vi "DS360 Receive Message.vi"(2 "timeout ms":u32=25000, 3 "address string":string, 4 "byte count":i32, 7 "source":string, 8 "read mode (EOI:0)":i32(ring)=2 items=["terminate read on EOI or byte count", "terminate read on EOI, byte count, or CR", "terminate read on EOI, byte count, or LF"], 9 "error in":T1) -> (0 "address out":string, 1 "read buffer":string, 5 "status":bool[](array[boolean]), 6 "error out":T1)   [LabVIEW 2025, in "MyDS360.lvlib"]
doc: "Sends a string to a message based VXI instrument. In order to communicate with an instrument, you must first open the instrument by running the Open VXI Instrument or running the initialize VI (initialize VIs call the Open VXI Instrument in their block diagram). Use the instrument ID generated by the Open VXI Instrument to address the specific instrument, then set the write mode and enter the string to send. If a write error occurs, error code 1230 is returned. If you fail to open the instrument, error code 1232 is returned."
uses:
  MyDS360.lvlib
panel:
  in  "[empty array]":bool[](array[boolean])
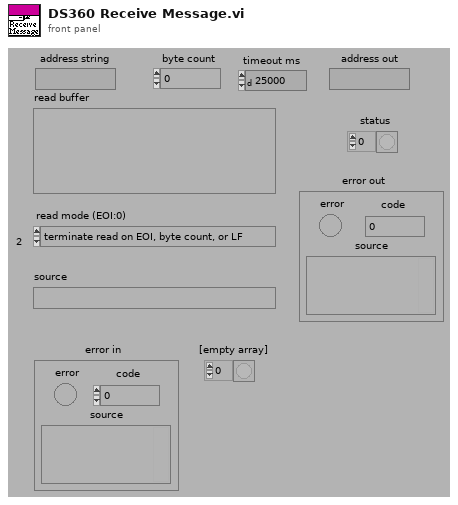
[diagram p1: front panel]
types:
  T1 = cluster{"error":bool, "code":i32, "source":string}
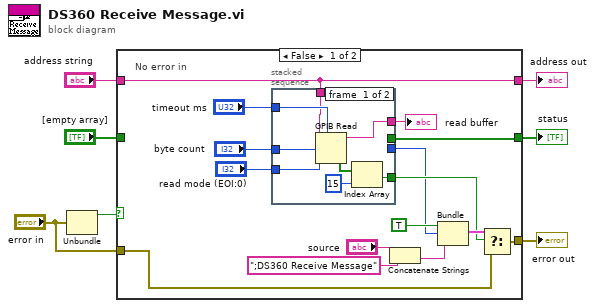
[diagram p0: block diagram]
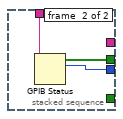
[diagram p2: hidden frame]
diagram:
  n1 = Unbundle("error in") -> ("error"=w5:bool)  [unwired: 2 out]
  n2 = case shown="False" w5 {
    tunnel: "[empty array]" -> [_ w35]
    tunnel: [w18 w35] -> w7
    tunnel: [w21 w36] -> w3
    tunnel: "error in" -> [w13 w36]
    tunnel: "address string" -> [w8 w34]
    tunnel: [w8 w34] -> w1
    frame False {
      # "No error in"
      n3 = stacked-sequence {
        tunnel: [_ w33] -> w18
        tunnel: [w28 _] -> w19
        tunnel: [_ w32] -> w17
        tunnel: "timeout ms" -> [w27 _]
        tunnel: "read mode (EOI:0)" -> [w26 _]
        tunnel: "byte count" -> [w25 _]
        tunnel: [w24 _] -> w9
        tunnel: w8 -> [w23 w31]
        frame #0 {
          n4 = GPIB Read(0:w23, 1:w25, 2:w26, 4:w27) -> (5:w24:string, 6:w29:bool[])  [unwired: 1 in, 1 out]
          n5 = Index Array(array=w29, index=15) -> (element=w28:bool)
        }
        frame #1 {
          n6 = GPIB Status(0:w31) -> (2:w33:bool[], 3:w32:i16)  [unwired: 1 in, 2 out]
        }
      }
      "read buffer" <- w9
      n7 = Concatenate Strings("source", ";DS360 Receive Message") -> (w14:string)
      n8 = Bundle(TRUE, "GPIB error"=w17, w14) -> (w22:cluster{bool, "GPIB error":i16, string})  [unwired: 1 in]
      n9 = Select(t=w22, s=w19, f=w13) -> (s? t:f=w21:T1)
    }
    frame True {
      # "Error in"
    }
  }
  "status" <- w7
  "error out" <- w3
  "address out" <- w1
